vi "FG JAUS Waypoints.vi"(1 "FG Action (Read)":T1, 2 "Waypoints In":T2[](array[typedef]) {"Longitude" format="%#_14g"; "Latitude" format="%#_14g"}) -> (0 "Waypoints Out":T2[](array[typedef]) {"Longitude" format="%#_14g"; "Latitude" format="%#_14g"})   [LabVIEW 2009]
uses:
  TypeDefs/Sensor TypeDefs/GPS Data.ctl
  cRIO/Functional Global Variables/Actions for FG's.ctl
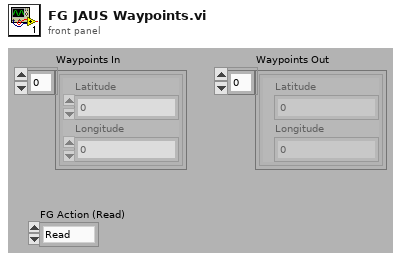
[diagram p1: front panel]
types:
  T1 = typedef "Actions for FG's.ctl" = enum16{"Read", "Write"}
  T2 = typedef "GPS Data.ctl" = cluster{"Latitude":dbl, "Longitude":dbl}
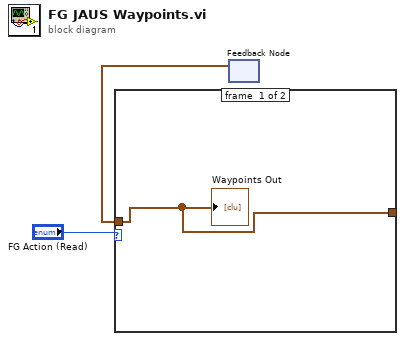
[diagram p0: block diagram]
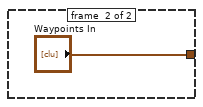
[diagram p2: hidden frame]
diagram:
  n1 = feedback #1() -> (w1:T2[])  [unwired: 1 in]
  n2 = case shown="\"Read\", Default" "FG Action (Read)" {
    tunnel: [w4 "Waypoints In"] -> w2
    tunnel: w1 -> [w4 _]
    frame #0 {
      "Waypoints Out" <- w4
    }
    frame #1 {
    }
  }
